vi "Configure Scan.vi"(0 "VISA resource name":refnum<visa-resource-name>, 1 "Settling Time (0)":dbl format="%#.6g", 2 "Enable 200V V-source Limit (T: Enable)":bool=TRUE, 5 "Scan Operation (2: None)":i32(ring)=2 items=["Internal", "External", "None"], 7 "External Scan Channels Number (10)":i32=10, 9 "Internal Scan List ((@ 1:10))":string="(@ 1:10)", 11 "error in (no error)":errorcluster, 12 "Switching Method (0: Voltage)":i32(ring) items=["Voltage", "Current"]) -> (4 "VISA resource name out":refnum<visa-resource-name>, 15 "error out":errorcluster)   [LabVIEW 2019, in "Keithley 6517.lvlib"]
doc: "Controls the 200V V-source limit, controls scan operation, internal scan or external scan, and configures settling time and switching method for internal scan.\n\n<B>Note:</B>\nThis VI is <B>NOT</B> compatible with model <B>6514</B>."
uses:
  Keithley 6517.lvlib
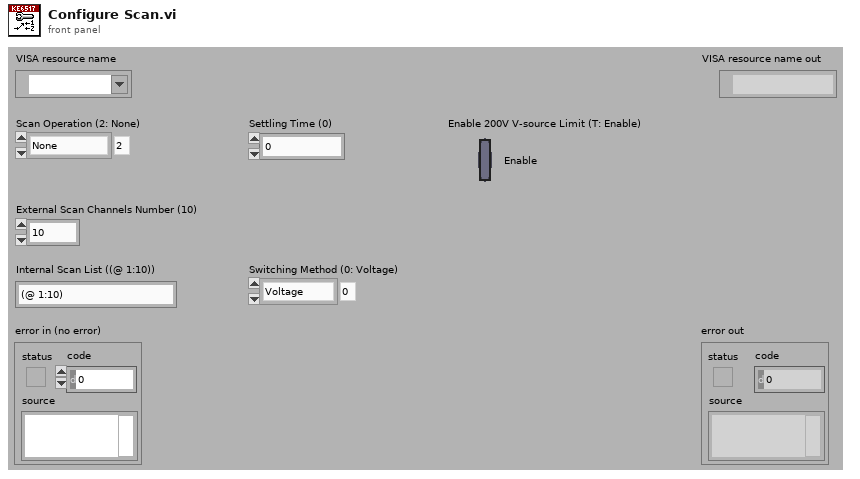
[diagram p1: front panel]
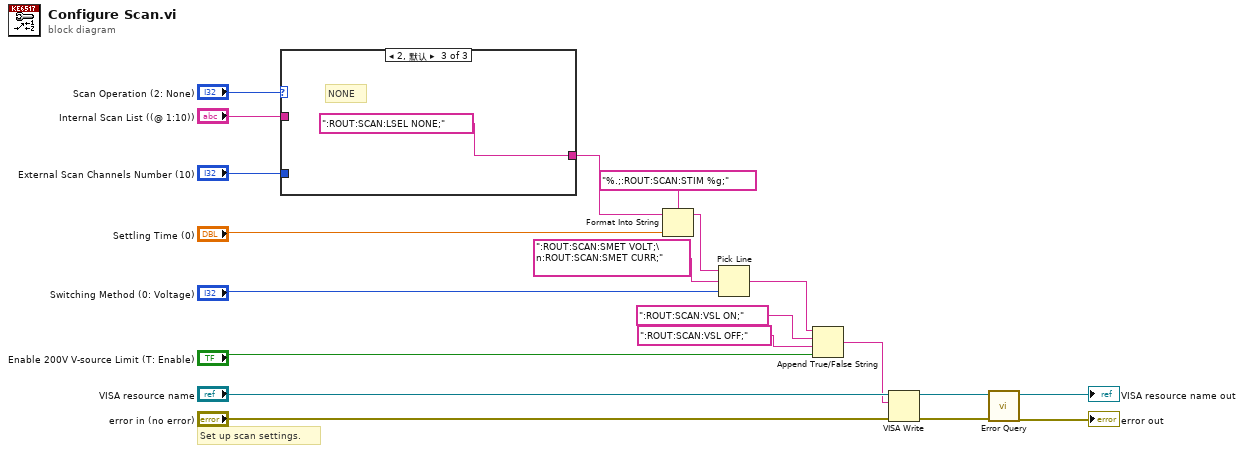
[diagram p0: block diagram]
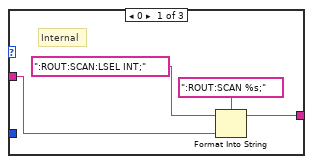
[diagram p2: hidden frame]
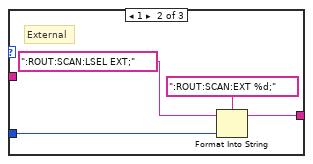
[diagram p3: hidden frame]
diagram:
  # "Set up scan settings."
  n1 = case shown="2, 默认" "Scan Operation (2: None)" {
    tunnel: "Internal Scan List ((@ 1:10))" -> [w22 _ _]
    tunnel: [w21 w26 ":ROUT:SCAN:LSEL NONE;"] -> w6
    tunnel: "External Scan Channels Number (10)" -> [_ w25 _]
    frame 0 {
      # "Internal"
      n2 = Format Into String(format string=":ROUT:SCAN %s;", initial string=":ROUT:SCAN:LSEL INT;", w22) -> (resulting string=w21:string)  [unwired: 1 in, 1 out]
    }
    frame 1 {
      # "External"
      n3 = Format Into String(format string=":ROUT:SCAN:EXT %d;", initial string=":ROUT:SCAN:LSEL EXT;", w25) -> (resulting string=w26:string)  [unwired: 1 in, 1 out]
    }
    frame 2, Default {
      # "NONE"
    }
  }
  n4 = Format Into String(format string="%.;:ROUT:SCAN:STIM %g;", initial string=w6, "Settling Time (0)") -> (resulting string=w7:string)  [unwired: 1 in, 1 out]
  n5 = Pick Line(string ("")=w7, multi-line string=":ROUT:SCAN:SMET VOLT;\n:ROUT:SCAN:SMET CURR;", line index="Switching Method (0: Voltage)") -> (output string=w8:string)
  n6 = Append True/False String(1:"Enable 200V V-source Limit (T: Enable)", 2:":ROUT:SCAN:VSL OFF;", 3:":ROUT:SCAN:VSL ON;", 4:w8) -> (0:w2:string)
  n7 = VISA Write(VISA resource name="VISA resource name", write buffer=w2, error in (no error)="error in (no error)") -> (VISA resource name out=w18:refnum<visa-resource-name>, error out=w17:errorcluster)  [unwired: 1 out]
  n8 = call "Error Query.vi"("error in (no error)"=w17, "VISA resource name"=w18) -> ("error out"=→"error out":errorcluster, "VISA resource name out"=→"VISA resource name out":refnum<visa-resource-name>)  [unwired: 6 in, 2 out]
